vi "Teleop.vi"(10 "Match Info":T1={"Autonomous Elapsed Seconds"=0.0, "TeleOp Elapsed Seconds"=0.0, "Disabled Elapsed Seconds"=0.0, "Visited Autonomous"=FALSE, "Visited TeleOp"=FALSE, "Visited Disabled"=FALSE, "Autonomous Settings"={"Autonomous Style"=enum."Independent", "VI Refnum"=refnum}}, 11 "Call Context":T2) -> ()   [LabVIEW 2020]
doc: "This VI is called for each TeleOp packet received from the DS where the robot is not disabled. It is often used to read from the joysticks and update I/O or to update setpoints for timed control loops. It should complete and return within 20 milliseconds or it may miss DS packets."
uses:
  <vilib>/Rock Robotics/WPI/DriverStation/WPI_DriverStationDerivedRobotMode.ctl
  <vilib>/Rock Robotics/WPI/DriverStation/WPI_DriverStationMatch Info.ctl
  <vilib>/Rock Robotics/WPI/Utilities/WPI_GetSetVariantRefNum.vi
  2017 Swerve Code/Swerve Global Variables.vi
  Robot Global Data.vi
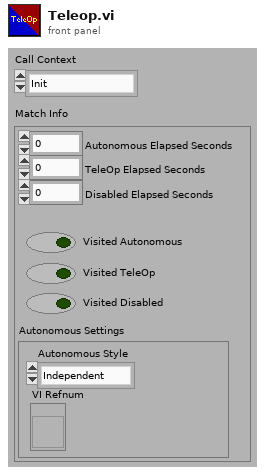
[diagram p1: front panel]
types:
  T1 = typedef "WPI_DriverStationMatch Info.ctl" = cluster{"Autonomous Elapsed Seconds":dbl, "TeleOp Elapsed Seconds":dbl, "Disabled Elapsed Seconds":dbl, "Visited Autonomous":bool, "Visited TeleOp":bool, "Visited Disabled":bool, "Autonomous Settings":cluster{"Autonomous Style":enum16{"Iterative", "Independent"}, "VI Refnum":refnum<vi>}}
  T2 = typedef "WPI_DriverStationDerivedRobotMode.ctl" = enum16{"Init", "Execute", "Stop"}
  T3 = typedef "WPI_JoystickDevRef.ctl" = cluster{"Device":T4}
  T4 = typedef "WPI_JoystickDeviceEnum.ctl" = enum16{"USB 0", "USB 1", "USB 2", "USB 3", "USB 4", "USB 5"}
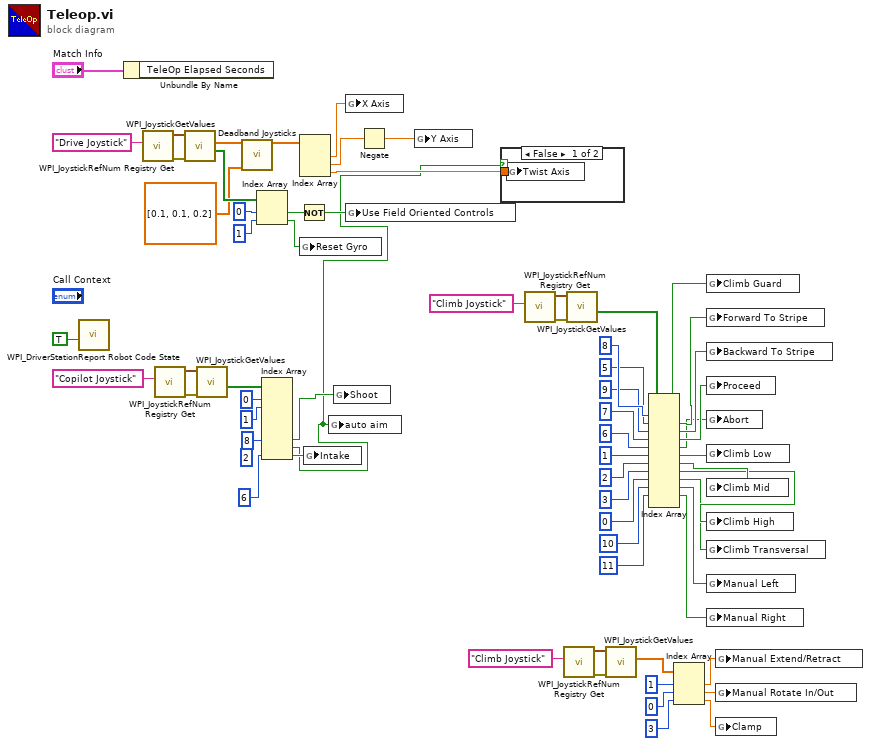
[diagram p0: block diagram]
diagram:
  (unwired) 2 ("index")
  n1 = call <vilib>:"WPI_DriverStationReport Robot Code State.vi"("TeleOp"=TRUE ("Autonomous")) -> ()  [unwired: 10 in, 1 out]
  n2 = Unbundle By Name("Match Info") -> ()  [unwired: 1 out]
  n3 = call <vilib>:"WPI_JoystickRefNum Registry Get.vi"("refnum name"="Drive Joystick") -> ("error out"=w53:errorcluster, "JoystickDevRef"=w63:T3)  [unwired: 1 in, 8 out]
  n4 = call <vilib>:"WPI_JoystickRefNum Registry Get.vi"("refnum name"="Copilot Joystick") -> ("error out"=w47:errorcluster, "JoystickDevRef"=w48:T3)  [unwired: 1 in, 8 out]
  n5 = call <vilib>:"WPI_JoystickGetValues.vi"("error in (no error)"=w53, "JoystickDevRef"=w63) -> ("Buttons"=w57:bool[], "Axes"=w52:dbl[])  [unwired: 5 in, 3 out]
  n6 = call <vilib>:"WPI_JoystickGetValues.vi"("error in (no error)"=w47, "JoystickDevRef"=w48) -> ("Buttons"=w46:bool[])  [unwired: 5 in, 4 out]
  n7 = call "Deadband Joysticks.vi"("Deadbands"=dbl[] [0.1, 0.1, 0.2], "Axes"=w52) -> ("Axes'"=w50:dbl[])  [unwired: 9 in]
  n8 = Index Array(array=w57, index #1=0 ("index"), index #2=1 ("index")) -> (element #1=w56:bool, element #2=w54:bool)
  n9 = Index Array(array=w46, index #1=0 ("index"), index #2=1 ("index"), index #7=8 ("index"), index #8=6 ("index")) -> (element #6=w38:bool, element #7=w37:bool, element #8=w40:bool)  [unwired: 4 in, 5 out]
  n10 = Not(x=w56) -> (.not. x?=w55:bool)
  n11 = Index Array(array=w50) -> (element #1=w61:dbl, element #2=w60:dbl, element #3=w59:dbl)  [unwired: 3 in]
  n12 = global write "Swerve Global Variables.vi" "Reset Gyro"(w54) -> ()
  n13 = global write "Robot Global Data.vi" "Intake"(w40) -> ()
  n14 = global write "Robot Global Data.vi" "auto aim"(w37) -> ()
  n15 = global write "Robot Global Data.vi" "Shoot"(w38) -> ()
  n16 = global write "Swerve Global Variables.vi" "X Axis"(w61) -> ()
  n17 = global write "Swerve Global Variables.vi" "Use Field Oriented Controls"(w55) -> ()
  n18 = Negate(x=w60) -> (-x=w58:dbl)
  n19 = global write "Swerve Global Variables.vi" "Y Axis"(w58) -> ()
  n20 = case shown="False" w37 {
    tunnel: w59 -> [w66 _]
    frame False {
      n21 = global write "Swerve Global Variables.vi" "Twist Axis"(w66) -> ()
    }
    frame True {
    }
  }
  n22 = call <vilib>:"WPI_JoystickRefNum Registry Get.vi"("refnum name"="Climb Joystick") -> ("error out"=w36:errorcluster, "JoystickDevRef"=w35:T3)  [unwired: 9 in]
  n23 = call <vilib>:"WPI_JoystickRefNum Registry Get.vi"("refnum name"="Climb Joystick") -> ("error out"=w33:errorcluster, "JoystickDevRef"=w32:T3)  [unwired: 9 in]
  n24 = call <vilib>:"WPI_JoystickGetValues.vi"("error in (no error)"=w36, "JoystickDevRef"=w35) -> ("Buttons"=w29:bool[])  [unwired: 5 in, 4 out]
  n25 = call <vilib>:"WPI_JoystickGetValues.vi"("error in (no error)"=w33, "JoystickDevRef"=w32) -> ("Axes"=w30:dbl[])  [unwired: 5 in, 4 out]
  n26 = Index Array(array=w29, index #1=8 ("index"), index #2=5 ("index"), index #3=9 ("index"), index #4=7 ("index"), index #5=6 ("index"), index #6=1 ("index"), index #7=2 ("index"), index #8=3 ("index"), index #9=0 ("index"), index #10=10 ("index"), index #11=11 ("index")) -> (element #1=w28:bool, element #2=w25:bool, element #3=w24:bool, element #4=w22:bool, element #5=w20:bool, element #6=w18:bool, element #7=w16:bool, element #8=w14:bool, element #9=w12:bool, element #10=w10:bool, element #11=w8:bool)  [unwired: 1 in, 1 out]
  n27 = Index Array(array=w30, index #1=1 ("index"), index #2=0 ("index"), index #3=3 ("index")) -> (element #1=w5:dbl, element #2=w4:dbl, element #3=w1:dbl)
  n28 = global write "Robot Global Data.vi" "Climb Guard"(w28) -> ()
  n29 = global write "Robot Global Data.vi" "Forward To Stripe"(w25) -> ()
  n30 = global write "Robot Global Data.vi" "Backward To Stripe"(w24) -> ()
  n31 = global write "Robot Global Data.vi" "Proceed"(w22) -> ()
  n32 = global write "Robot Global Data.vi" "Abort"(w20) -> ()
  n33 = global write "Robot Global Data.vi" "Climb Low"(w18) -> ()
  n34 = global write "Robot Global Data.vi" "Climb Mid"(w16) -> ()
  n35 = global write "Robot Global Data.vi" "Climb High"(w14) -> ()
  n36 = global write "Robot Global Data.vi" "Climb Transversal"(w12) -> ()
  n37 = global write "Robot Global Data.vi" "Manual Left"(w10) -> ()
  n38 = global write "Robot Global Data.vi" "Manual Right"(w8) -> ()
  n39 = global write "Swerve Global Variables.vi" "Manual Extend/Retract"(w5) -> ()
  n40 = global write "Swerve Global Variables.vi" "Manual Rotate In/Out"(w4) -> ()
  n41 = global write "Swerve Global Variables.vi" "Clamp"(w1) -> ()
